vi "5_ВПДелениеНаНоль.vi"() -> ()   [LabVIEW 2016]
panel:
  out "Ошибка!":bool
  out "Результат":dbl
  out "Случайное число-делимое":dbl
  in  "Делитель":dbl
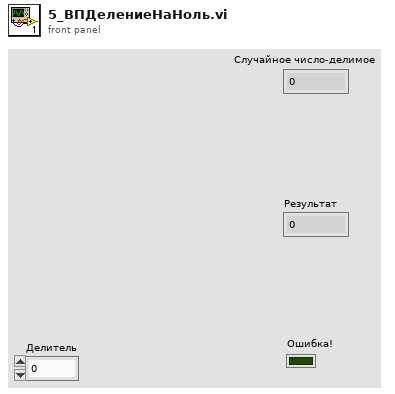
[diagram p1: front panel]
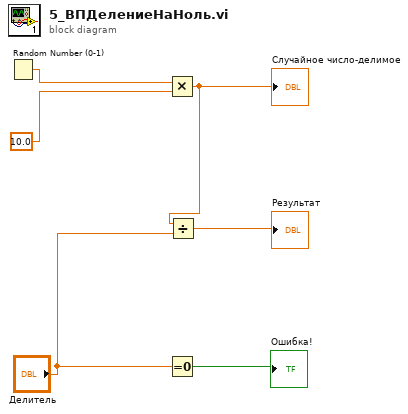
[diagram p0: block diagram]
diagram:
  n1 = Random Number (0-1)() -> (number: 0 to 1=w3:dbl)
  n2 = Multiply(x=w3, y=10.0) -> (x*y=w4:dbl)
  "Случайное число-делимое" <- w4
  n3 = Equal To 0?(x="Делитель") -> (x = 0?=→"Ошибка!":bool)
  n4 = Divide(x=w4, y="Делитель") -> (x/y=→"Результат":dbl)
